vi "rad_degree.vi"(1 "Boolean":bool, 2 "rad/degree":dbl) -> (0 "degree/rad":dbl)   [LabVIEW 2016]
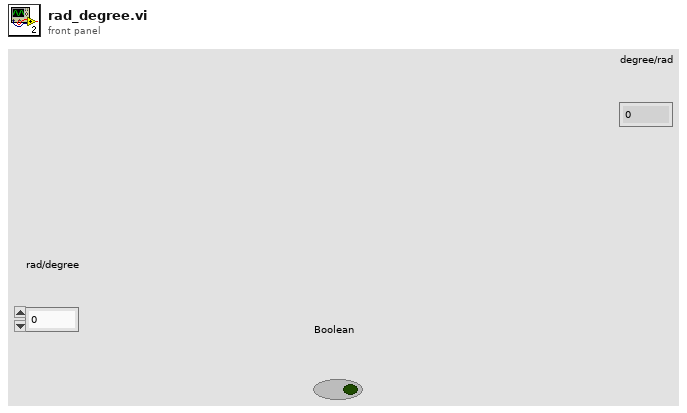
[diagram p1: front panel]
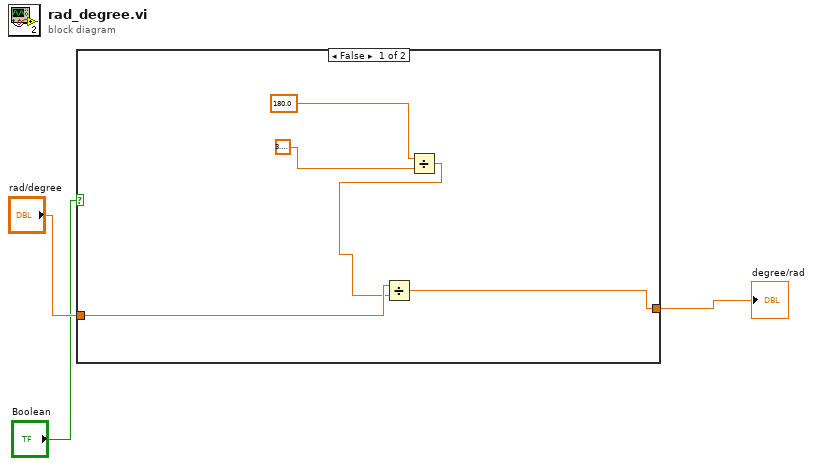
[diagram p0: block diagram]
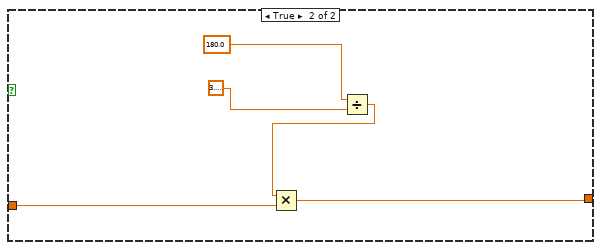
[diagram p2: hidden frame]
diagram:
  n1 = case shown="False" "Boolean" {
    tunnel: "rad/degree" -> [w6 w11]
    tunnel: [w4 w9] -> w1
    frame False {
      n2 = Divide(x=180.0 ("y"), y=3.141592653589793) -> (x/y=w5:dbl)
      n3 = Divide(x=w6, y=w5) -> (x/y=w4:dbl)
    }
    frame True {
      n4 = Divide(x=180.0 ("y"), y=3.141592653589793) -> (x/y=w10:dbl)
      n5 = Multiply(x=w10, y=w11) -> (x*y=w9:dbl)
    }
  }
  "degree/rad" <- w1
